vi "HardwareLoop.vi"(8 "Error In":errorcluster, 9 "Executable Configuration":T2, 10 "Data Structures":T1, 11 "Action Queues":T3) -> (0 "Error Out":errorcluster)   [LabVIEW 2012]
uses:
  ActionQueues.ctl
  UIActionQueueElement.ctl
  UIAction.ctl
  HardwareActionQueueElement.ctl
  HardwareAction.ctl
  LogActionQueueElement.ctl
  LogAction.ctl
  ExecutableConfiguration.ctl
  DataStructures.ctl
  HardwareDisplayData.ctl
  HardwareLogData.ctl
  SetupGlobalAction.ctl
  HardwareAbortGlobalAction.ctl
  <vilib>/Utility/error.llb/DialogType.ctl
  driver/Keithley-2602.lvlib
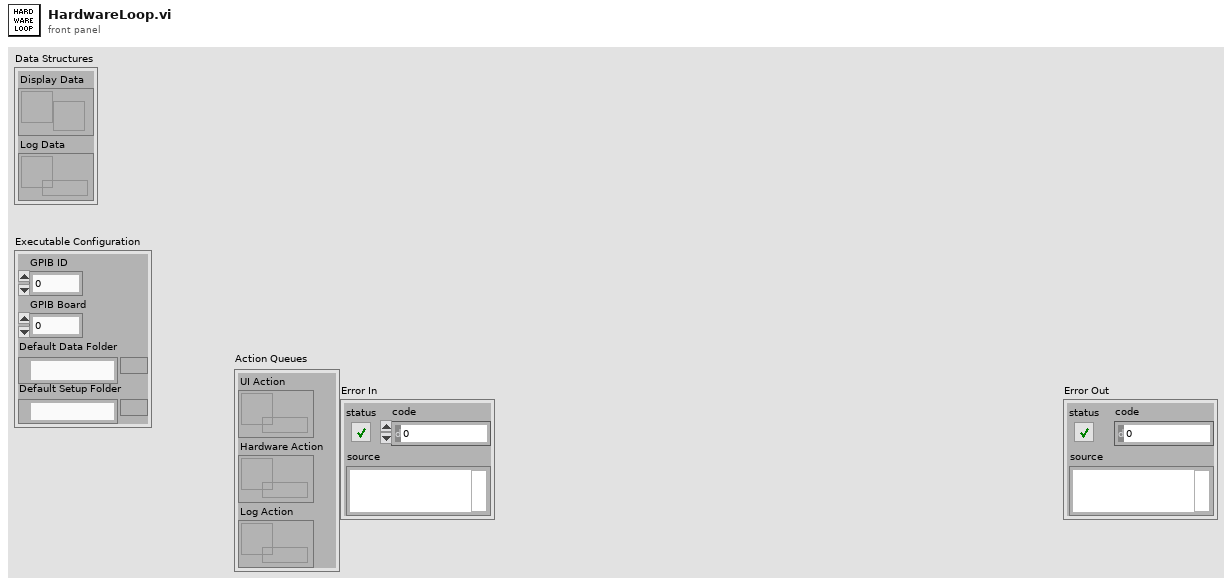
[diagram p1: front panel]
types:
  T1 = typedef "DataStructures.ctl" = cluster{"Display Data":refnum<notifier>, "Log Data":refnum<queue>}
  T2 = typedef "ExecutableConfiguration.ctl" = cluster{"GPIB ID":u8, "GPIB Board":u8, "Default Data Folder":path, "Default Setup Folder":path}
  T3 = typedef "ActionQueues.ctl" = cluster{"UI Action":refnum<queue>, "Hardware Action":refnum<queue>, "Log Action":refnum<queue>}
  T4 = typedef "HardwareActionQueueElement.ctl" = cluster{"Action":T5, "Data":variant}
  T5 = typedef "HardwareAction.ctl" = enum16{"Initialize", "Start", "Run", "Stop", "Error", "Shutdown"}
  T6 = typedef "SetupGlobalAction.ctl" = enum16{"Get", "Set", "Reset"}
  T7 = typedef "UIActionQueueElement.ctl" = cluster{"Action":T8, "Data":variant}
  T8 = typedef "UIAction.ctl" = enum16{"Initialize", "Configure Trigger", "Configure Measure", "Configure Source", "Configure DUT", "Configure Log", "Configure Open", "Configure Save", "Configure Reset", "Hardware Start", "Hardware Started", "Hardware Stop", "Hardware Stopped", "Log Arm", "Log Start", "Log Started", "Log Stop", "Log Stopped", "Create Chart", "Error", "Shutdown"}
  T9 = typedef "HardwareLogData.ctl" = cluster{"Timestamp":timestamp, "Data":T10}
  T10 = typedef "HardwareDisplayData.ctl" = cluster{"DUT Names":string[][], "SMU":dbl[][], "Port":bool[]}
  T11 = typedef "HardwareAbortGlobalAction.ctl" = enum16{"Set", "Get"}
  T12 = typedef "Setup.ctl" = cluster{"DUT":T13, "Log":T15, "Trigger":T23, "Sources":T29[], "Measures":T31[]}
  T13 = typedef "DUTConfiguration.ctl" = cluster{"Count":u32, "Wirings":T14[], "Names":string[][]}
  T14 = typedef "Keithley-2602.lvlib/SMUSense.ctl" = enum16{"Local (2-wire)", "Remote (4-wire)", "Calibration"}
  T15 = typedef "LogConfiguration.ctl" = cluster{"Start":T16, "Rollover":T19, "Stop":T21}
  T16 = typedef "LogStartConfiguration.ctl" = cluster{"Trigger Type":T17, "Timer (sec)":dbl, "Digital IO Line":u8, "Digital IO Edge":T18}
  T17 = typedef "LogStartTriggerType.ctl" = enum16{"Immediate", "User", "Timer", "Digital IO"}
  T18 = typedef "LogDigitalIOTriggerEdge.ctl" = enum16{"Rising", "Falling"}
  T19 = typedef "LogRolloverConfiguration.ctl" = cluster{"Trigger Type":T20, "Timer (sec)":dbl, "File Size (MB)":u32, "Digital IO Line":u8, "Digital IO Edge":T18}
  T20 = typedef "LogRolloverTriggerType.ctl" = enum16{"None", "Timer", "File Size", "Digital IO"}
  T21 = typedef "LogStopConfiguration.ctl" = cluster{"Trigger Type":T22, "Timer (sec)":dbl, "File Size (MB)":u32, "Digital IO Line":u8, "Digital IO Edge":T18}
  T22 = typedef "LogStopTriggerType.ctl" = enum16{"None", "User", "Timer", "File Size", "Digital IO"}
  T23 = typedef "TriggerConfiguration.ctl" = cluster{"Input":T24, "Output":T27}
  T24 = typedef "TriggerInputConfiguration.ctl" = cluster{"Type":T25, "Timeout (ms)":u32, "Delay (ms)":u32, "Digital IO Line (1-14)":u8, "Digital IO Mode":T26}
  T25 = typedef "TriggerInputType.ctl" = enum16{"None", "Digital IO", "Bus"}
  T26 = typedef "Keithley-2602.lvlib/TriggerMode.ctl" = enum16{"Falling", "Rising", "Either", "Synchronous"}
  T27 = typedef "TriggerOutputConfiguration.ctl" = cluster{"Type":T28, "Delay (ms)":u32, "Digital IO Line (1-14)":u8, "Digital IO Mode":T26, "Digital IO Pulse Width (sec)":dbl}
  T28 = typedef "TriggerOutputType.ctl" = enum16{"None", "Digital IO", "Bus"}
  T29 = typedef "SourceConfiguration.ctl" = cluster{"Enabled?":bool, "Function":T30, "Level (V or A)":dbl, "Autorange Enabled?":bool, "High Limit (V or A)":dbl, "Low Limit (V or A)":dbl}
  T30 = typedef "SourceFunction.ctl" = enum16{"Voltage", "Current"}
  T31 = typedef "MeasureConfiguration.ctl" = cluster{"Enabled?":bool, "Count":u8, "Interval (sec)":dbl, "Voltage Auto Range Enabled?":bool, "Voltage High Limit (V or A)":dbl, "Voltage Low Limit (V or A)":dbl, "Current Auto Range Enabled?":bool, "Current High Limit (V or A)":dbl, "Current Low Limit (V or A)":dbl}
  T32 = typedef "DialogType.ctl" = u16
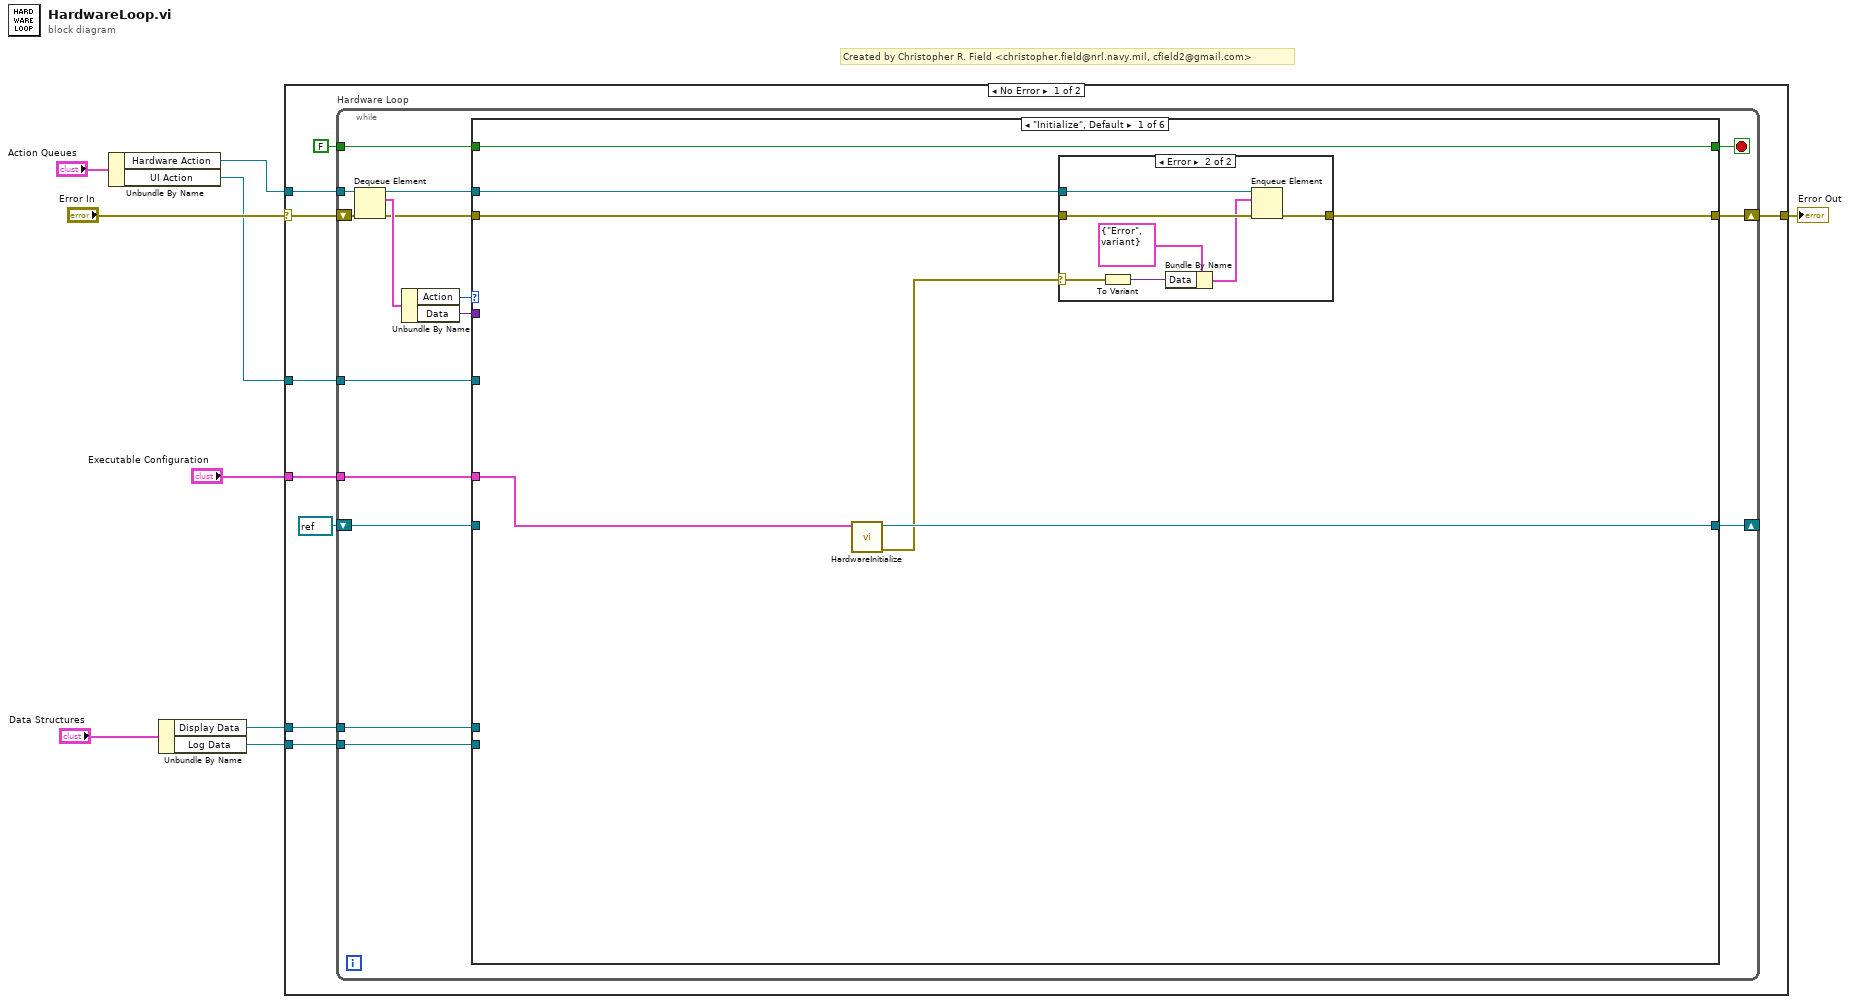
[diagram p0: block diagram]
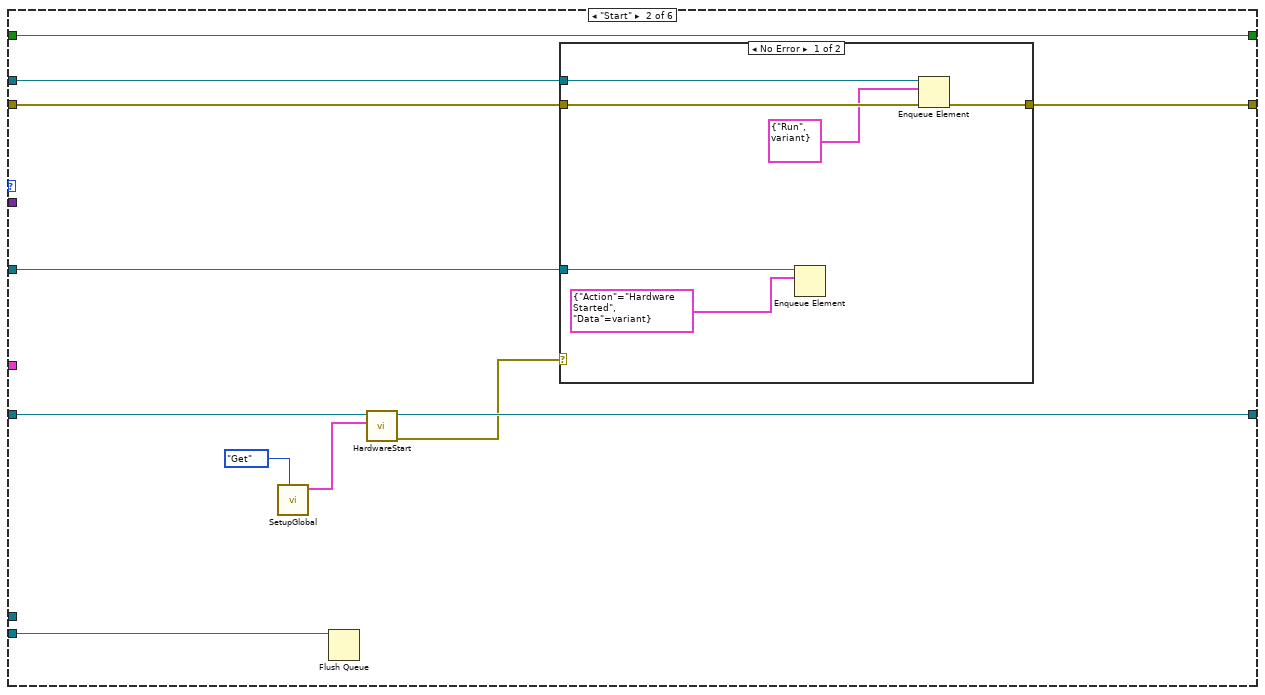
[diagram p3: hidden frame]
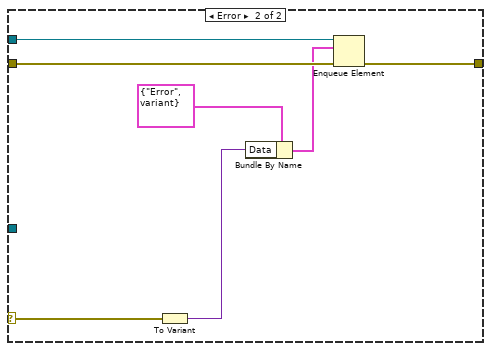
[diagram p4: hidden frame]
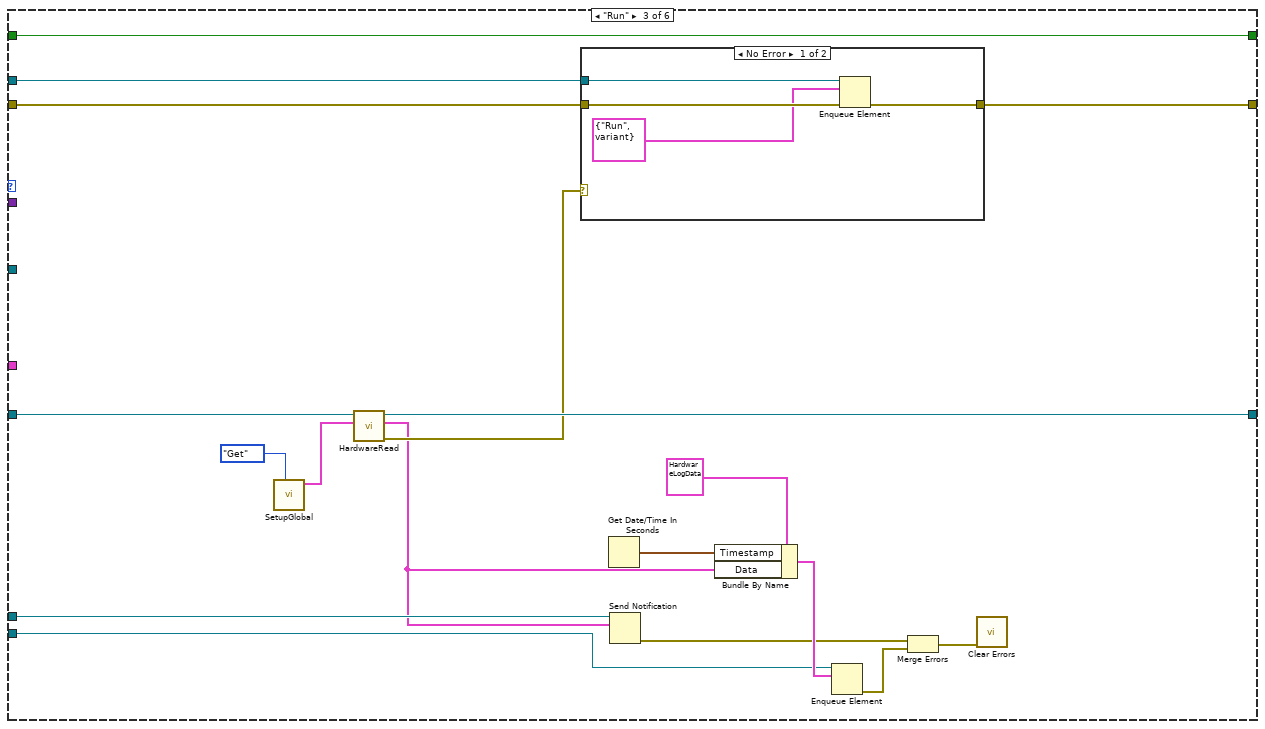
[diagram p5: hidden frame]
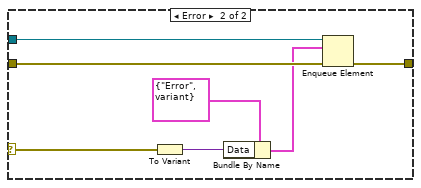
[diagram p6: hidden frame]
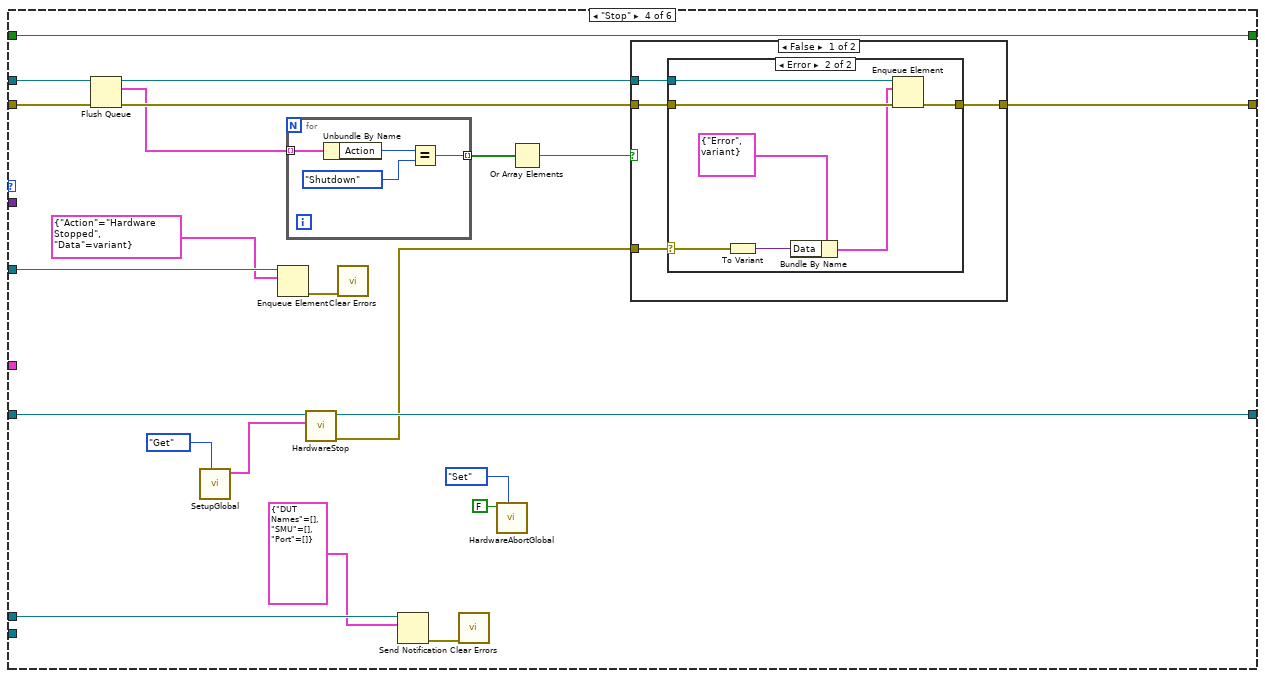
[diagram p7: hidden frame]
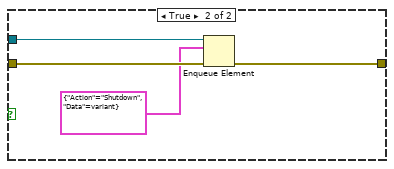
[diagram p9: hidden frame]
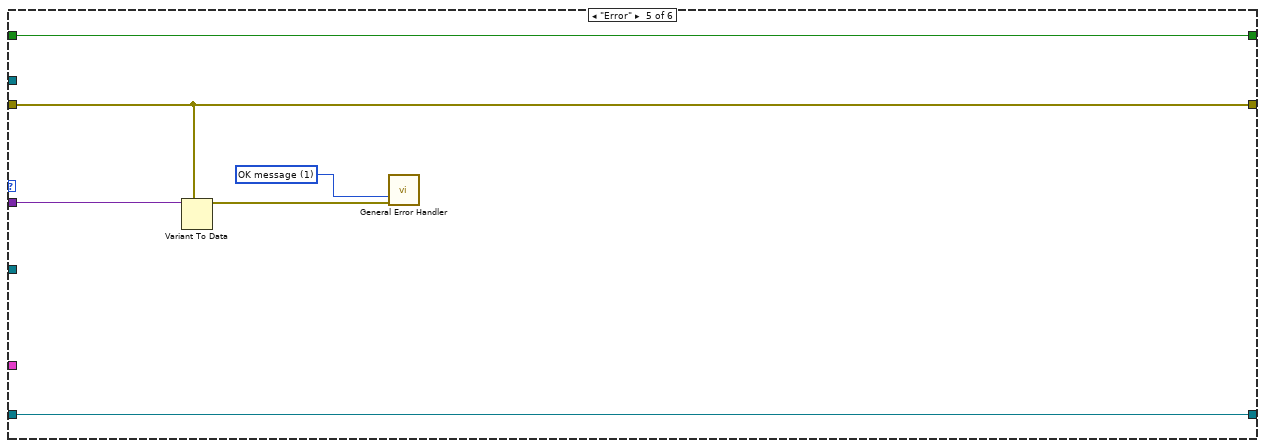
[diagram p10: hidden frame]
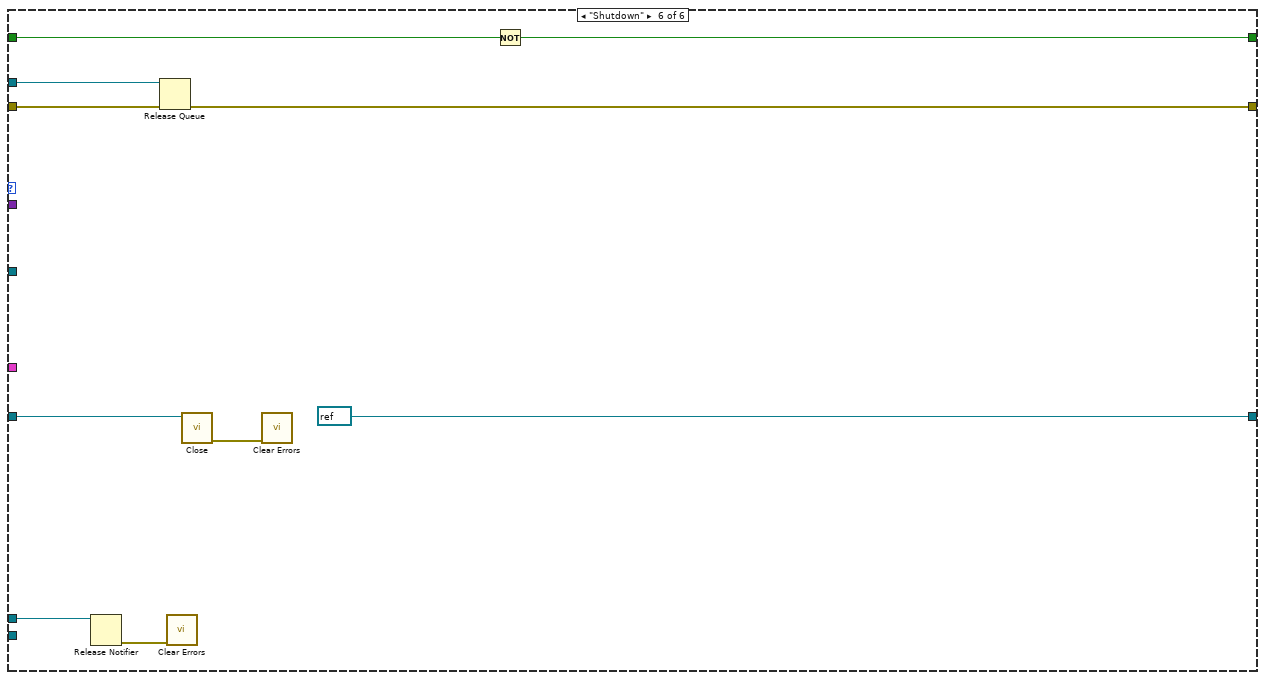
[diagram p11: hidden frame]
diagram:
  # "Created by Christopher R. Field <christopher.field@nrl.navy.mil, cfield2@gmail.com>"
  n1 = Unbundle By Name("Action Queues") -> ("Hardware Action"=w8:refnum<queue>, "UI Action"=w1:refnum<queue>)
  n2 = Unbundle By Name("Data Structures") -> ("Display Data"=w3:refnum<notifier>, "Log Data"=w2:refnum<queue>)
  n3 = case shown="No Error" "Error In" {
    selector: "Error In" -> [w17 w161]
    tunnel: w8 -> [w18 _]
    tunnel: [w15 w161] -> w6
    tunnel: "Executable Configuration" -> [w14 _]
    tunnel: w3 -> [w12 _]
    tunnel: w2 -> [w11 _]
    tunnel: w1 -> [w10 _]
    frame No Error {
      n4 = while "Hardware Loop" {
        tunnel: w18 -> [w34]
        shift-right: [w25] -> w15
        shift-left: w17 -> [w33]
        tunnel: FALSE -> [w27]
        tunnel: w14 -> [w24]
        shift-right: [w23] -> _
        shift-left: refnum<visa-resource-name> refnum ("Keithley 2602 Out") -> [w22]
        tunnel: w12 -> [w21]
        tunnel: w11 -> [w20]
        tunnel: w10 -> [w19]
        stop <- w26 stop-if-true
        n5 = Dequeue Element(queue=w34, error in (no error)=w33) -> (queue out=w28:refnum<queue>, element=w32:T4, error out=w29:errorcluster)  [unwired: 1 in, 1 out]
        n6 = Unbundle By Name(w32) -> ("Action"=w31:T5, "Data"=w30:variant)
        n7 = case shown="\"Initialize\", Default" w31 {
          tunnel: w30 -> [_ _ _ _ w148 _]
          tunnel: w29 -> [w37 w56 w86 w110 w147 w157]
          tunnel: w28 -> [w40 w55 w87 w111 _ w158]
          tunnel: w27 -> [w41 w60 w91 w124 w150 w160]
          tunnel: [w41 w60 w91 w124 w150 w159] -> w26
          tunnel: [w39 w54 w85 w120 w147 w156] -> w25
          tunnel: w24 -> [w38 _ _ _ _ _]
          tunnel: [w36 w58 w89 w122 w149 refnum<visa-resource-name> refnum ("Keithley 2602 Out")] -> w23
          tunnel: w22 -> [_ w59 w90 w123 w149 w155]
          tunnel: w21 -> [_ _ w84 w117 _ w152]
          tunnel: w20 -> [_ w52 w80 _ _ _]
          tunnel: w19 -> [_ w53 _ w119 _ _]
          frame "Initialize", Default {
            n8 = call "HardwareInitialize.vi"("Executable Configuration"=w38) -> ("Error Out"=w35:errorcluster, "Keithley 2602 Out"=w36:refnum<visa-resource-name>)  [unwired: 9 in]
            n9 = case shown="Error" w35 {
              selector: w35 -> [_ w44]
              tunnel: w37 -> [w42 w48]
              tunnel: w40 -> [_ w49]
              tunnel: [w42 w47] -> w39
              frame No Error {
              }
              frame Error {
                n10 = To Variant(anything=w44) -> (Variant=w45:variant)
                n11 = Bundle By Name(cluster=T4 {"Action"=enum."Error", "Data"=variant} ("element"), "Data"=w45) -> (w43:T4)
                n12 = Enqueue Element(queue=w49, element=w43, error in (no error)=w48) -> (error out=w47:errorcluster)  [unwired: 1 in, 2 out]
              }
            }
          }
          frame "Start" {
            n13 = call "SetupGlobal.vi"("Action"=SetupGlobalAction."Get") -> ("Value Out"=w50:T12)  [unwired: 10 in]
            n14 = Flush Queue(queue=w52) -> ()  [unwired: 1 in, 3 out]
            n15 = call "HardwareStart.vi"("Setup"=w50, "Keithley 2602 In"=w59) -> ("Error Out"=w57:errorcluster, "Keithley 2602 Out"=w58:refnum<visa-resource-name>)  [unwired: 8 in]
            n16 = case shown="No Error" w57 {
              selector: w57 -> [_ w68]
              tunnel: w56 -> [w65 w72]
              tunnel: w55 -> [w66 w73]
              tunnel: [w64 w71] -> w54
              tunnel: w53 -> [w62 _]
              frame No Error {
                n17 = Enqueue Element(queue=w62, element=T7 {"Action"=enum."Hardware Started", "Data"=variant}) -> ()  [unwired: 2 in, 3 out]
                n18 = Enqueue Element(queue=w66, element=T4 {"Action"=enum."Run", "Data"=variant}, error in (no error)=w65) -> (error out=w64:errorcluster)  [unwired: 1 in, 2 out]
              }
              frame Error {
                n19 = To Variant(anything=w68) -> (Variant=w69:variant)
                n20 = Bundle By Name(cluster=T4 {"Action"=enum."Error", "Data"=variant} ("element"), "Data"=w69) -> (w67:T4)
                n21 = Enqueue Element(queue=w73, element=w67, error in (no error)=w72) -> (error out=w71:errorcluster)  [unwired: 1 in, 2 out]
              }
            }
          }
          frame "Run" {
            n22 = call "SetupGlobal.vi"("Action"=SetupGlobalAction."Get") -> ("Value Out"=w74:T12)  [unwired: 10 in]
            n23 = call "HardwareRead.vi"("Setup"=w74, "Keithley 2602 In"=w90) -> ("Error Out"=w88:errorcluster, "Hardware Display Data"=w79:T10, "Keithley 2602 Out"=w89:refnum<visa-resource-name>)  [unwired: 7 in]
            n24 = case shown="No Error" w88 {
              selector: w88 -> [_ w97]
              tunnel: w87 -> [w95 w102]
              tunnel: w86 -> [w94 w101]
              tunnel: [w93 w100] -> w85
              frame No Error {
                n25 = Enqueue Element(queue=w95, element=T4 {"Action"=enum."Run", "Data"=variant}, error in (no error)=w94) -> (error out=w93:errorcluster)  [unwired: 1 in, 2 out]
              }
              frame Error {
                n26 = To Variant(anything=w97) -> (Variant=w98:variant)
                n27 = Bundle By Name(cluster=T4 {"Action"=enum."Error", "Data"=variant} ("element"), "Data"=w98) -> (w96:T4)
                n28 = Enqueue Element(queue=w102, element=w96, error in (no error)=w101) -> (error out=w100:errorcluster)  [unwired: 1 in, 2 out]
              }
            }
            n29 = Get Date/Time In Seconds() -> (seconds since 1Jan1904=w82:timestamp)
            n30 = Send Notification(notification=w79, notifier=w84) -> (error out=w78:errorcluster)  [unwired: 1 in, 1 out]
            n31 = Bundle By Name(cluster=T9 {"Timestamp"=timestamp(0 s since 1904-01-01), "Data"={"DUT Names"=[], "SMU"=[], "Port"=[]}} ("Hardware Log Data"), "Timestamp"=w82, "Data"=w79) -> (w81:T9)
            n32 = Enqueue Element(queue=w80, element=w81) -> (error out=w77:errorcluster)  [unwired: 2 in, 2 out]
            n33 = Merge Errors(w78, w77) -> (w76:errorcluster)
            n34 = call <vilib>:"Clear Errors.vi"("error in (no error)"=w76) -> ()  [unwired: 6 in, 1 out]
          }
          frame "Stop" {
            n35 = Flush Queue(queue=w111, error in (no error)=w110) -> (queue out=w108:refnum<queue>, remaining elements=w107:T4[], error out=w109:errorcluster)
            n36 = call "SetupGlobal.vi"("Action"=SetupGlobalAction."Get") -> ("Value Out"=w103:T12)  [unwired: 10 in]
            n37 = Enqueue Element(queue=w119, element=T7 {"Action"=enum."Hardware Stopped", "Data"=variant}) -> (error out=w115:errorcluster)  [unwired: 2 in, 2 out]
            n38 = for {
              tunnel: w107 -> [w144] mode=indexing
              tunnel: [w141] -> w106 mode=indexing
              n39 = Unbundle By Name(w144) -> ("Action"=w143:T5)
              n40 = Equal?(x=w143, y=HardwareAction."Shutdown") -> (x = y?=w141:bool)
            }
            n41 = call "HardwareStop.vi"("Setup"=w103, "Keithley 2602 In"=w123) -> ("Error Out"=w121:errorcluster, "Keithley 2602 Out"=w122:refnum<visa-resource-name>)  [unwired: 8 in]
            n42 = call <vilib>:"Clear Errors.vi"("error in (no error)"=w115) -> ()  [unwired: 6 in, 1 out]
            n43 = Send Notification(notification=T10 {"DUT Names"=[], "SMU"=[], "Port"=[]}, notifier=w117) -> (error out=w114:errorcluster)  [unwired: 1 in, 1 out]
            n44 = call <vilib>:"Clear Errors.vi"("error in (no error)"=w114) -> ()  [unwired: 6 in, 1 out]
            n45 = call "HardwareAbortGlobal.vi"("Action"=HardwareAbortGlobalAction."Set", "Set Value"=FALSE) -> ()  [unwired: 9 in, 1 out]
            n46 = Or Array Elements(Boolean array=w106) -> (logical OR=w105:bool)
            n47 = case shown="False" w105 {
              tunnel: w121 -> [w128 _]
              tunnel: [w127 w138] -> w120
              tunnel: w109 -> [w126 w139]
              tunnel: w108 -> [w125 w140]
              frame False {
                n48 = case shown="Error" w128 {
                  selector: w128 -> [_ w132]
                  tunnel: w126 -> [w129 w135]
                  tunnel: w125 -> [_ w136]
                  tunnel: [w129 w130] -> w127
                  frame No Error {
                  }
                  frame Error {
                    n49 = To Variant(anything=w132) -> (Variant=w133:variant)
                    n50 = Bundle By Name(cluster=T4 {"Action"=enum."Error", "Data"=variant} ("element"), "Data"=w133) -> (w131:T4)
                    n51 = Enqueue Element(queue=w136, element=w131, error in (no error)=w135) -> (error out=w130:errorcluster)  [unwired: 1 in, 2 out]
                  }
                }
              }
              frame True {
                n52 = Enqueue Element(queue=w140, element=T4 {"Action"=enum."Shutdown", "Data"=variant}, error in (no error)=w139) -> (error out=w138:errorcluster)  [unwired: 1 in, 2 out]
              }
            }
          }
          frame "Error" {
            w145 = T32 1 items=["no dialog", "OK message", "continue or stop message", "OK message + warnings", "continue/stop + warnings"] ("type of dialog (OK msg:1)")
            n53 = Variant To Data(type=w147, Variant=w148) -> (data=w146:errorcluster)  [unwired: 1 in, 1 out]
            n54 = call <vilib>:"General Error Handler.vi"("type of dialog (OK msg:1)"=w145, "error in (no error)"=w146) -> ()  [unwired: 9 in, 5 out]
          }
          frame "Shutdown" {
            n55 = Release Notifier(notifier=w152) -> (error out=w151:errorcluster)  [unwired: 2 in, 2 out]
            n56 = Release Queue(queue=w158, error in (no error)=w157) -> (error out=w156:errorcluster)  [unwired: 1 in, 2 out]
            n57 = call <vilib>:"Clear Errors.vi"("error in (no error)"=w151) -> ()  [unwired: 6 in, 1 out]
            n58 = call "Close.vi"("Keithley 2602 In"=w155) -> ("Error Out"=w154:errorcluster)  [unwired: 10 in]
            n59 = call <vilib>:"Clear Errors.vi"("error in (no error)"=w154) -> ()  [unwired: 6 in, 1 out]
            n60 = Not(x=w160) -> (.not. x?=w159:bool)
          }
        }
      }
    }
    frame Error {
    }
  }
  "Error Out" <- w6
